vi "calc_variables.vi"(6 "var2":dbl, 7 "Peletron":dbl, 8 "var1":dbl, 9 "Mass":dbl[](array[numeric]), 10 "Charge":dbl[](array[numeric]), 11 "Velocity":dbl[](array[numeric])) -> (1 "Mass out":dbl[](array[numeric]), 2 "Charge out":dbl[](array[numeric]), 3 "Velocity out":dbl[](array[numeric]))   [LabVIEW 2012]
uses:
  <vilib>/Analysis/Matrix/Datatypes/RealMatrix.ctl
  <vilib>/Analysis/Matrix/NI_Matrix.lvlib
panel:
  out "appended array":T1
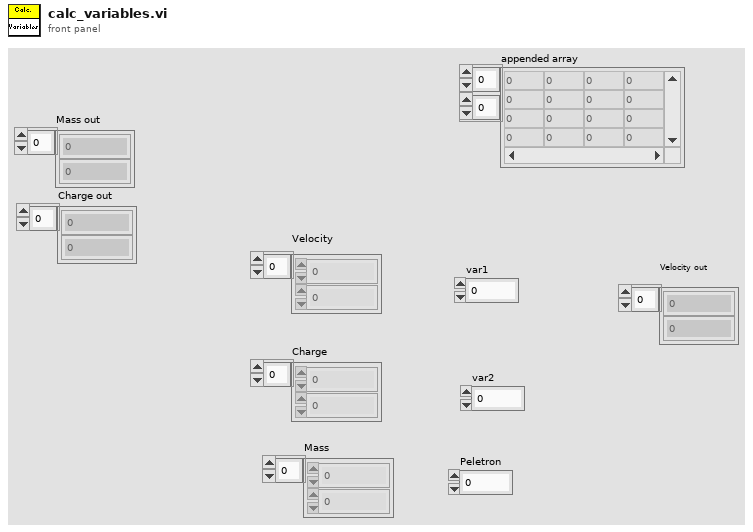
[diagram p1: front panel]
types:
  T1 = typedef "NI_Matrix.lvlib/RealMatrix.ctl" = dbl[][]
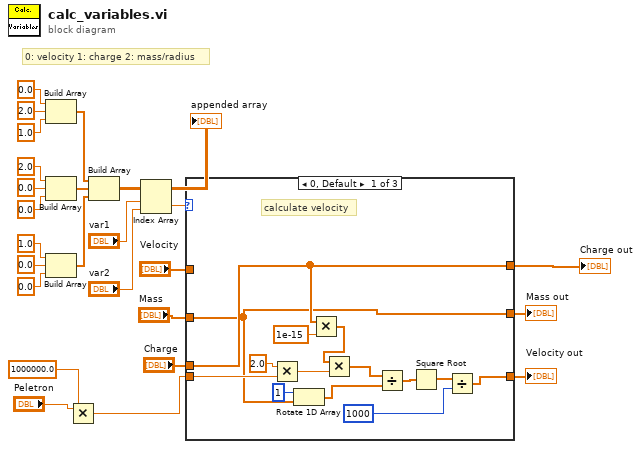
[diagram p0: block diagram]
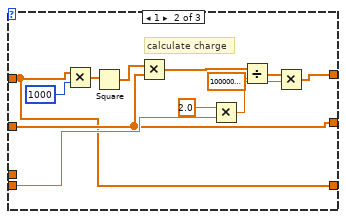
[diagram p2: hidden frame]
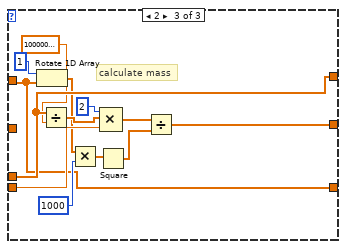
[diagram p3: hidden frame]
diagram:
  # "0: velocity 1: charge 2: mass/radius"
  n1 = Build Array(0.0 ("element"), 2.0 ("element"), 1.0 ("element")) -> (w16:dbl[])
  n2 = Build Array(2.0 ("element"), 0.0 ("element"), 0.0 ("element")) -> (w15:dbl[])
  n3 = Build Array(1.0 ("element"), 0.0 ("element"), 0.0 ("element")) -> (w14:dbl[])
  n4 = Multiply(x="Peletron", y=1000000.0) -> (x*y=w1:dbl)
  n5 = Build Array(w16, w15, w14) -> (w13:T1)
  "appended array" <- w13
  n6 = Index Array(array=w13, index (row)="var1", index (col)="var2") -> (element=w10:dbl)
  n7 = case shown="0, Default" w10 {
    tunnel: "Velocity" -> [_ w43 w52]
    tunnel: "Mass" -> [w26 w46 _]
    tunnel: "Charge" -> [w34 _ w59]
    tunnel: w1 -> [w38 w50 w63]
    tunnel: [w29 w43 w52] -> w6
    tunnel: [w26 w46 w60] -> w5
    tunnel: [w34 w40 w59] -> w4
    frame 0, Default {
      # "calculate velocity"
      n8 = Multiply(x=2.0, y=w38) -> (x*y=w37:dbl)
      n9 = Rotate 1D Array(1:w26, 2:1 ("n")) -> (0:w27:dbl[])
      n10 = Multiply(x=w34, y=1e-15) -> (x*y=w32:dbl[])
      n11 = Multiply(x=w32, y=w37) -> (x*y=w36:dbl[])
      n12 = Divide(x=w36, y=w27) -> (x/y=w35:dbl[])
      n13 = Square Root(x=w35) -> (sqrt(x)=w31:dbl[])
      n14 = Divide(x=w31, y=1000) -> (x/y=w29:dbl[])
    }
    frame 1 {
      # "calculate charge"
      n15 = Multiply(x=w43, y=1000) -> (x*y=w44:dbl[])
      n16 = Square(x=w44) -> (x^2=w49:dbl[])
      n17 = Multiply(x=w49, y=w46) -> (x*y=w48:dbl[])
      n18 = Multiply(x=2.0, y=w50) -> (x*y=w47:dbl)
      n19 = Divide(x=w48, y=w47) -> (x/y=w42:dbl[])
      n20 = Multiply(x=w42, y=1000000000000000.0) -> (x*y=w40:dbl[])
    }
    frame 2 {
      # "calculate mass"
      n21 = Rotate 1D Array(1:w52, 2:1 ("n")) -> (0:w53:dbl[])
      n22 = Divide(x=w59, y=1000000000000000.0) -> (x/y=w58:dbl[])
      n23 = Multiply(x=w53, y=1000) -> (x*y=w56:dbl[])
      n24 = Square(x=w56) -> (x^2=w61:dbl[])
      n25 = Compound Arithmetic op=MULTIPLY(2, w58, w63) -> (w62:dbl[])
      n26 = Divide(x=w62, y=w61) -> (x/y=w60:dbl[])
    }
  }
  "Velocity out" <- w6
  "Mass out" <- w5
  "Charge out" <- w4
